vi "Read trusted entities.vi"(8 "error in (no error)":errorcluster, 11 "Connection.TCP-TLS in":refnum<class "Connection.TCP-TLS.lvclass">) -> (0 "error out":errorcluster, 2 "trusted entities":path[](array[path]), 3 "Connection.TCP-TLS out":refnum<class "Connection.TCP-TLS.lvclass">)   [LabVIEW 2020, in "Connection.TCP-TLS.lvclass"]
uses:
  Connection.TCP-TLS.lvclass
  Connection.TCP-TLS.lvclass/Connection.TCP-TLS.ctl
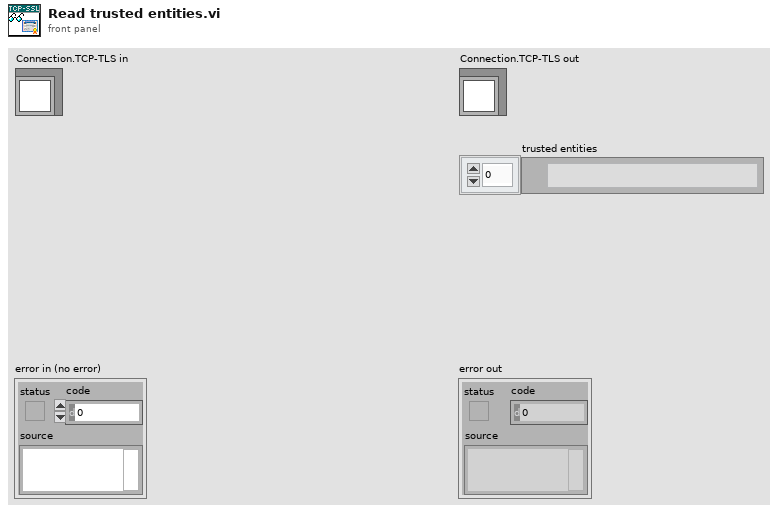
[diagram p1: front panel]
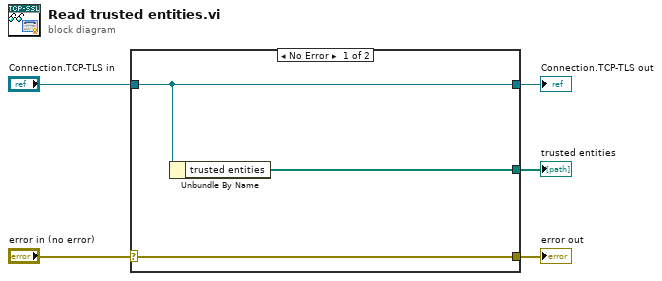
[diagram p0: block diagram]
diagram:
  n1 = case shown="No Error" "error in (no error)" {
    selector: "error in (no error)" -> [w8 w9]
    tunnel: [w8 w9] -> w4
    tunnel: [w7 w10] -> w2
    tunnel: "Connection.TCP-TLS in" -> [w7 w10]
    tunnel: [w6 _] -> w1
    frame No Error {
      n2 = Unbundle By Name(w7) -> ("trusted entities"=w6:path[])
    }
    frame Error {
    }
  }
  "error out" <- w4
  "Connection.TCP-TLS out" <- w2
  "trusted entities" <- w1
